vi "FTP_dir.vi"(0 "connection ID":refnum<k5>, 2 "error in":errorcluster) -> (3 "connection ID out":refnum<k5>, 4 "reply string":string, 5 "Good Reply?":bool, 6 "error out":errorcluster)   [LabVIEW 2012]
panel:
  out "directory listing":string
  in  "chunk size (4096)":i32=4096
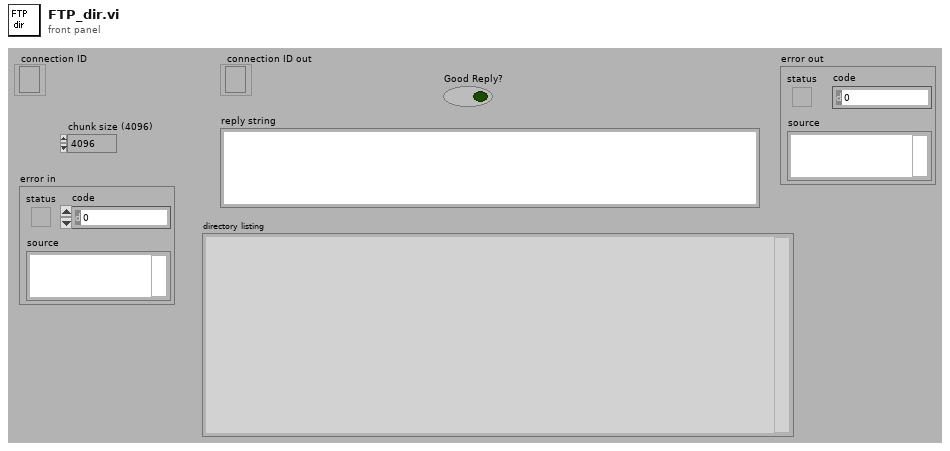
[diagram p1: front panel]
types:
  T1 = enum16{"unknown", "100 + Prelim", "200 + ", "300 + Intermed", "400 - Transient", "500 - Permanent"}
  T2 = cluster{"passive address":string, "passive port":u16}
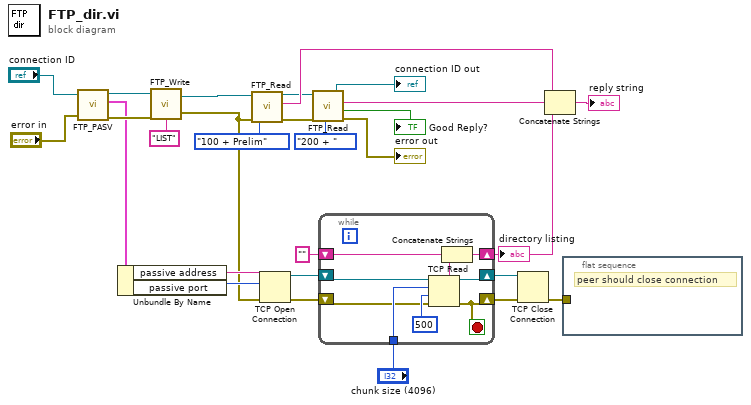
[diagram p0: block diagram]
diagram:
  n1 = call <userlib>:"FTP_PASV.vi"("connection ID"="connection ID", "error in"="error in") -> ("connection ID out"=w23:refnum<k5>, "Passive Port"=w15:T2, "error out"=w22:errorcluster)  [unwired: 2 out]
  n2 = Unbundle By Name(w15) -> ("passive address"=w16:string, "passive port"=w17:u16)
  n3 = call <userlib>:"FTP_Write.vi"("Cmd"="LIST", "error in"=w22, "connection ID in"=w23) -> ("error out"=w8:errorcluster, "connection ID out"=w26:refnum<k5>)  [unwired: 1 in]
  n4 = call <userlib>:"FTP_Read.vi"("error In"=w8, "expected class"=T1."100 + Prelim", "connection ID"=w26) -> ("error out"=w6:errorcluster, "reply string"=w11:string, "connection ID out"=w7:refnum<k5>)  [unwired: 2 out]
  n5 = TCP Open Connection(address=w16, remote port or service name=w17, error in (no error)=w8) -> (connection ID=w18:refnum<k5>, error out=w19:errorcluster)  [unwired: 2 out]
  n6 = call <userlib>:"FTP_Read.vi"("error In"=w6, "expected class"=T1."200 + ", "connection ID"=w7) -> ("error out"=→"error out":errorcluster, "Good Reply?"=→"Good Reply?":bool, "reply string"=w1:string, "connection ID out"=→"connection ID out":refnum<k5>)  [unwired: 1 out]
  n7 = while {
    shift-right: [w33] -> w21
    shift-left: w18 -> [w35]
    shift-right: [w29] -> w20
    shift-left: w19 -> [w34]
    tunnel: "chunk size (4096)" -> [w36]
    shift-right: [w30] -> w10
    shift-left: "" -> [w32]
    stop <- w29 stop-if-true
    n8 = TCP Read(connection ID=w35, bytes to read=w36, error in (no error)=w34, 9:500 ("timeout ms (25000)")) -> (connection ID out=w33:refnum<k5>, data out=w31:string, error out=w29:errorcluster)  [unwired: 1 out]
    n9 = Concatenate Strings(w32, w31) -> (w30:string)
  }
  "directory listing" <- w10
  n10 = TCP Close Connection(connection ID=w21, error in (no error)=w20) -> (error out=w12:errorcluster)  [unwired: 2 out]
  n11 = Concatenate Strings(w11, w1, w10) -> (→"reply string":string)
  n12 = flat-sequence {
    tunnel: w12 -> [_]
    frame #0 {
      # "peer should close connection"
    }
  }
